vi "DAQ configuration.vi"() -> (3 "data":dynamicdata(waveform))   [LabVIEW 2025]
panel:
  in  "data 2":dbl
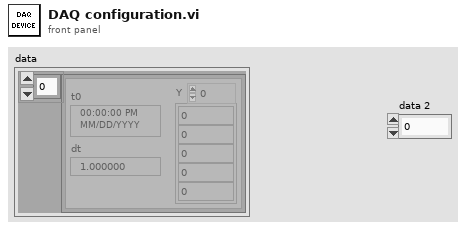
[diagram p1: front panel]
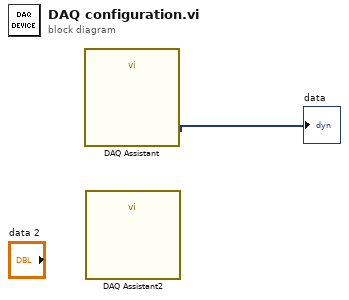
[diagram p0: block diagram]
diagram:
  n1 = call "DAQ Assistant"() -> ("data"=→"data":dynamicdata)  [unwired: 17 in, 2 out]
  n2 = call "DAQ Assistant2"() -> ()  [unwired: 18 in, 2 out]
